vi "XGT 결과 읽기.vi"(8 "error in (no error)":errorcluster, 11 "VISA resource name":refnum<visa-resource-name>="COM4" caption="VISA 리소스 이름") -> (0 "error out":errorcluster, 2 "appended array":string[](array[string]), 3 "VISA Refnum out":refnum<visa-resource-name>, 4 "응답":string="\u00060ARSB016400000000000000000000000000000000000000000000000000000000000000000000000000000000000000000000000000000000000000000000000000000000000000000000000000000000000000000000000000000000000000000000000000000000\u0003")   [LabVIEW 2014]
uses:
  <vilib>/regexp/Match Regular Expression.xnode
panel:
  out "데이터":string
  out "Header 잘라내기":string
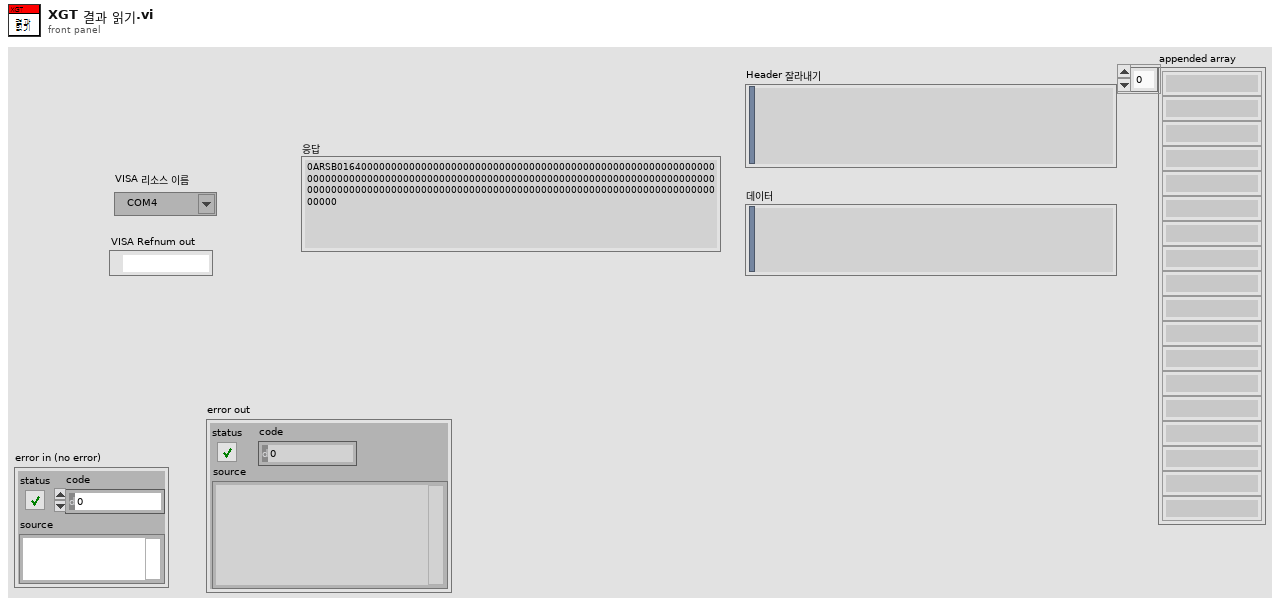
[diagram p1: front panel]
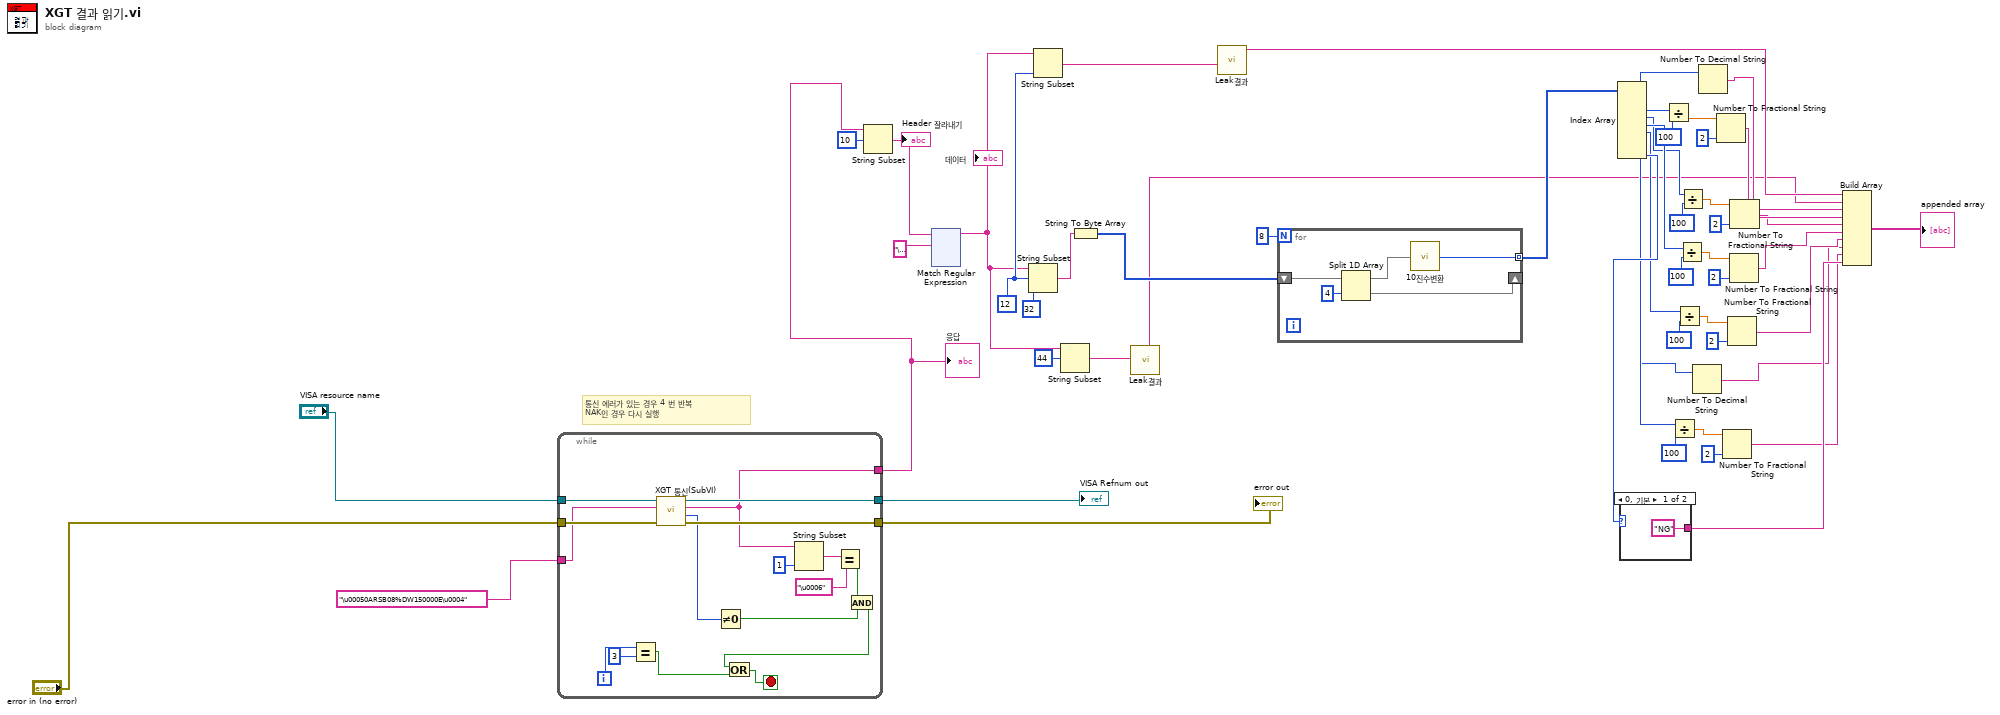
[diagram p0: block diagram]
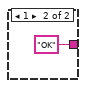
[diagram p2: hidden frame]
diagram:
  w9 = 12 ("offset (0)")
  # "통신 에러가 있는 경우 4 번 반복\nNAK인 경우 다시 실행"
  n1 = while {
    tunnel: "VISA resource name" -> [w70]
    tunnel: "error in (no error)" -> [w69]
    tunnel: [w68] -> w53
    tunnel: [w67] -> w1
    tunnel: "\u00050ARSB08%DW150000E\u0004" -> [w54]
    tunnel: [w55] -> w45
    i -> [w66]
    stop <- w64 stop-if-true
    n2 = Equal?(x=w66, y=3) -> (x = y?=w63:bool)
    n3 = call "XGT 통신(SubVI).vi"("error in (no error)"=w69, "String"=w54, "VISA Refnum in"=w70) -> ("error out"=w67:errorcluster, "Bytes at Port"=w62:u32, "read buffer"=w55:string, "VISA Refnum out"=w68:refnum<visa-resource-name>)  [unwired: 5 in]
    n4 = Not Equal To 0?(x=w62) -> (x != 0?=w57:bool)
    n5 = String Subset(string=w55, length (rest)=1 ("length (rest)")) -> (substring=w60:string)  [unwired: 1 in]
    n6 = Equal?(x=w60, y="\u0006") -> (x = y?=w58:bool)
    n7 = And(x=w58, y=w57) -> (x .and. y?=w56:bool)
    n8 = Or(x=w56, y=w63) -> (x .or. y?=w64:bool)
  }
  "error out" <- w1
  "응답" <- w45
  "VISA Refnum out" <- w53
  n9 = String Subset(string=w45, offset (0)=10 ("오프셋(0)")) -> (substring=w48:string)  [unwired: 1 in]
  "Header 잘라내기" <- w48
  n10 = xnode "Match Regular Expression"("입력 문자열"=w48, "정규식"="\u0003") -> ("일치 구문 앞"=w2:string)  [unwired: 4 in, 4 out]
  "데이터" <- w2
  n11 = String Subset(string=w2, offset (0)=w9, length (rest)=32 ("length (rest)")) -> (substring=w3:string)
  n12 = String Subset(string=w2, length (rest)=w9) -> (substring=w43:string)  [unwired: 1 in]
  n13 = String Subset(string=w2, offset (0)=44) -> (substring=w6:string)  [unwired: 1 in]
  n14 = String To Byte Array(string=w3) -> (unsigned byte array=w46:u8[])
  n15 = call "Leak결과.vi"("일치 구문 앞"=w6) -> ("String"=w4:string)  [unwired: 10 in]
  n16 = call "Leak결과.vi"("일치 구문 앞"=w43) -> ("String"=w5:string)  [unwired: 10 in]
  n17 = for {
    N: 8 -> [_]
    shift-right: [w73] -> _
    shift-left: w46 -> [w75]
    tunnel: [w71] -> w42 mode=indexing
    n18 = Split 1D Array(array=w75, index=4 ("인덱스")) -> (first subarray=w72:u8[], second subarray=w73:u8[])
    n19 = call "10진수변환.vi"("16진수"=w72) -> ("숫자형"=w71:i32)
  }
  n20 = Index Array(array=w42) -> (element #1=w38:i32, element #2=w41:i32, element #3=w13:i32, element #4=w32:i32, element #5=w28:i32, element #6=w11:i32, element #7=w24:i32, element #8=w39:i32)  [unwired: 8 in]
  n21 = case shown="0, 기본" w39 {
    tunnel: ["NG" "OK"] -> w21
    frame 0, Default {
    }
    frame 1 {
    }
  }
  n22 = Divide(x=w41, y=100) -> (x/y=w37:dbl)
  n23 = Divide(x=w24, y=100) -> (x/y=w26:dbl)
  n24 = Divide(x=w28, y=100) -> (x/y=w30:dbl)
  n25 = Divide(x=w32, y=100) -> (x/y=w34:dbl)
  n26 = Divide(x=w13, y=100) -> (x/y=w15:dbl)
  n27 = Number To Decimal String(number=w11) -> (decimal integer string=w10:string)  [unwired: 1 in]
  n28 = Number To Decimal String(number=w38) -> (decimal integer string=w23:string)  [unwired: 1 in]
  n29 = Number To Fractional String(number=w37, precision (6)=i16 2) -> (F-format string=w22:string)  [unwired: 2 in]
  n30 = Number To Fractional String(number=w26, precision (6)=i16 2) -> (F-format string=w17:string)  [unwired: 2 in]
  n31 = Number To Fractional String(number=w30, precision (6)=i16 2) -> (F-format string=w18:string)  [unwired: 2 in]
  n32 = Number To Fractional String(number=w34, precision (6)=i16 2) -> (F-format string=w19:string)  [unwired: 2 in]
  n33 = Number To Fractional String(number=w15, precision (6)=i16 2) -> (F-format string=w12:string)  [unwired: 2 in]
  n34 = Build Array(w5, w4, w23, w22, w12, w19, w18, w10, w17, w21) -> (→"appended array":string[])
